vi "Create Table LVClass.vi"(0 "PDF Report":refnum<class "PDF Report Class.lvclass">, 1 "Repeat Headers Row":bool=TRUE, 2 "Table columnWidth [ ]":sgl[](array[numeric]), 3 "Table type":T1, 5 "Column Headers 2D [ ]":string[][](array[string]), 7 "Row Headers 1D [ ]":string[](array[string]), 9 "Text Data 2D [ ]":string[][](array[string]), 11 "error in (no error)":errorcluster, 12 "Image to Add [ ]":T2 {"Scale" format="%#_g %"}) -> (4 "PDF Report duplicate":refnum<class "PDF Report Class.lvclass">, 8 "PDF Table":refnum<class "Pdfp Table Class.lvclass">, 15 "error out":errorcluster)   [LabVIEW 2019]
doc: "Version 2.0\nDeveloped by Jean-Marc Simard\nCopyright © 2012, Exaprom Inc.\nAll rights reserved.\nLicense: BSD\n\nWith iTextSharp 4.1.6 (http://itextsharp.sourceforge.net)\nunder Mozilla Public License Version 1.1\n(http://www.mozilla.org/MPL/MPL-1.1.html)"
uses:
  <userlib>/Exaprom PDF/Controls/General Controls/Image to Add [ ].ctl
  <userlib>/Exaprom PDF/Controls/Image Controls/Image Scale.ctl
  <userlib>/Exaprom PDF/LV Class/Pdfp Table Class/Pdfp Table Class.lvclass
  <userlib>/Exaprom PDF/LV Class/PDF Report Class/PDF Report Class.lvclass
  <userlib>/Exaprom PDF/Controls/Table Controls/Table type.ctl
  <userlib>/Exaprom PDF/Controls/Table Controls/Table Custom Titles or data.ctl
  <userlib>/Exaprom PDF/Controls/Table Controls/Table Custom type Titles or Datas.ctl
  <userlib>/Exaprom PDF/Controls/Table Controls/Cell Border iText number.ctl
  <userlib>/Exaprom PDF/Controls/Font Controls/Font complete B.ctl
  <userlib>/Exaprom PDF/Controls/Font Controls/Font size.ctl
  <userlib>/Exaprom PDF/Controls/Font Controls/Font color.ctl
  <userlib>/Exaprom PDF/Controls/Text Controls/Texte alignement.ctl
  <userlib>/Exaprom PDF/Controls/Table Controls/Cell Vertical alignment.ctl
  <userlib>/Exaprom PDF/Controls/Text Controls/Line spacing.ctl
  <userlib>/Exaprom PDF/Controls/Text Controls/Unicode/ASCII or Unicode with Select.ctl
  <userlib>/Exaprom PDF/Controls/Text Controls/Unicode/Character type with Select.ctl
  <userlib>/Exaprom PDF/Controls/Text Controls/Unicode/Writing direction with Select.ctl
  <userlib>/Exaprom PDF/LV Class/Fonts Class/Font Class.lvclass
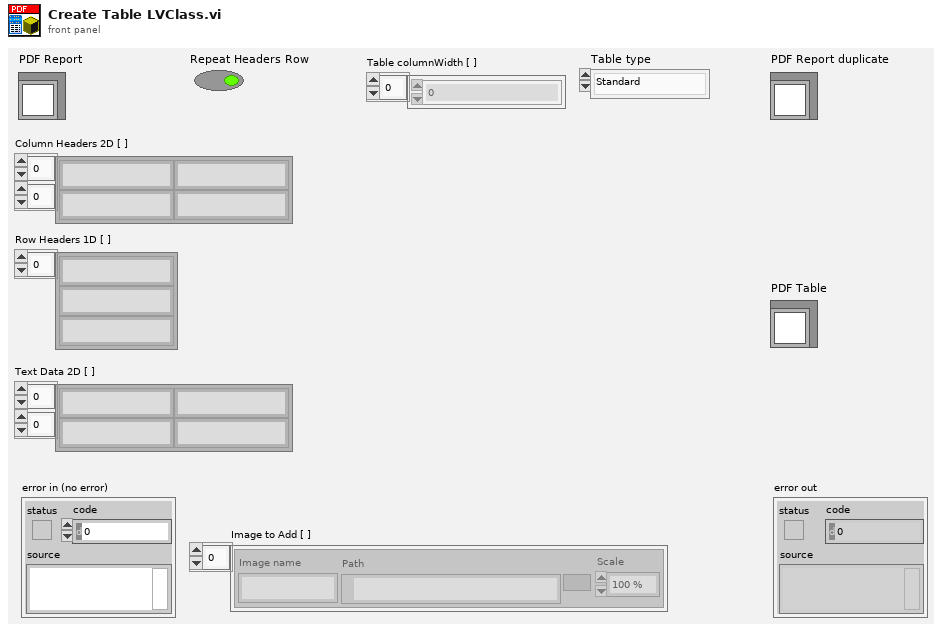
[diagram p1: front panel]
types:
  T1 = typedef "Table type.ctl" = enum16{"Standard", "Customized"}
  T2 = typedef "Image to Add [ ].ctl" = cluster{"Image name":string, "Path":path, "Scale":T3}[]
  T3 = typedef "Image Scale.ctl" = sgl
  T4 = typedef "Table Custom Titles or data.ctl" = cluster{"Titles or datas":T5, "Repeat on each new page?":bool, "Row":cluster{"#":i16, "to #":i16}, "Table columnWidth [ ]":sgl[], "Merge [ ]":cluster{"from":i8, "to":i8}[], "Cell [ ]":cluster{"Cluster 2":cluster{"Cell Border":T6, "Line":cluster{"Thickness":sgl, "Color":u32}, "BG":u32}, "Font":T7, "Align. and LS":cluster{"Horizontal":T10, "Vertical":T11, "Line spacing":T12}}[], "Text 2D":string[][], "ASCII or Unicode":T13}
  T5 = typedef "Table Custom type Titles or Datas.ctl" = enum16{"Title", "Data"}
  T6 = typedef "Cell Border iText number.ctl" = u16
  T7 = typedef "Font complete B.ctl" = cluster{"Name":string, "Size":T8, "Color":T9, "Style":cluster{"Bold":bool, "Italic":bool, "Underline":bool, "Strikeout":bool}, "Embed":bool, "Encoding":string}
  T8 = typedef "Font size.ctl" = sgl
  T9 = typedef "Font color.ctl" = u32
  T10 = typedef "Texte alignement.ctl" = enum16{"Select", "CENTER", "JUSTIFY", "LEFT", "RIGHT"}
  T11 = typedef "Cell Vertical alignment.ctl" = enum16{"TOP", "MIDDLE", "BOTTOM"}
  T12 = typedef "Line spacing.ctl" = enum16{"Select", "1.0", "1.5", "2.0"}
  T13 = typedef "ASCII or Unicode with Select.ctl" = cluster{"Type":T14, "Direction":T15}
  T14 = typedef "Character type with Select.ctl" = enum16{"Select", "ASCII", "Unicode"}
  T15 = typedef "Writing direction with Select.ctl" = enum16{"Select", "Default", "NO BIDI", "LTR", "RTL"}
  T16 = typedef "Font complete cluster.ctl" = cluster{"Name":string, "Size":T8, "Color":T9, "Style":cluster{"Bold":bool, "Italic":bool, "Underline":bool, "Strikeout":bool}, "Type":T17}
  T17 = typedef "Type and encoding.ctl" = cluster{"Type&direction":T18, "Embedded":bool, "Encoding":string}
  T18 = typedef "Type and run direction.ctl" = enum16{"Select", "ASCII", "UTF-16", "UTF-16 (default)", "UTF-16 (LTR)", "UTF-16 (RTL)"}
  T19 = typedef "System Fonts.ctl" = cluster{"Font name [ ]":string[], "Font and file names [ ]":cluster{"Font name":string, "File name":string}[]}
  T20 = typedef "Defaut Paragraphe and Line Spacing.ctl" = cluster{" Aligment":T10, "Line spacing":T12}
  T21 = cluster{"Paragraphe cluster":T20, "Font OUT":T16, "Font Ref":refnum<k24>, "System Fonts":T19}
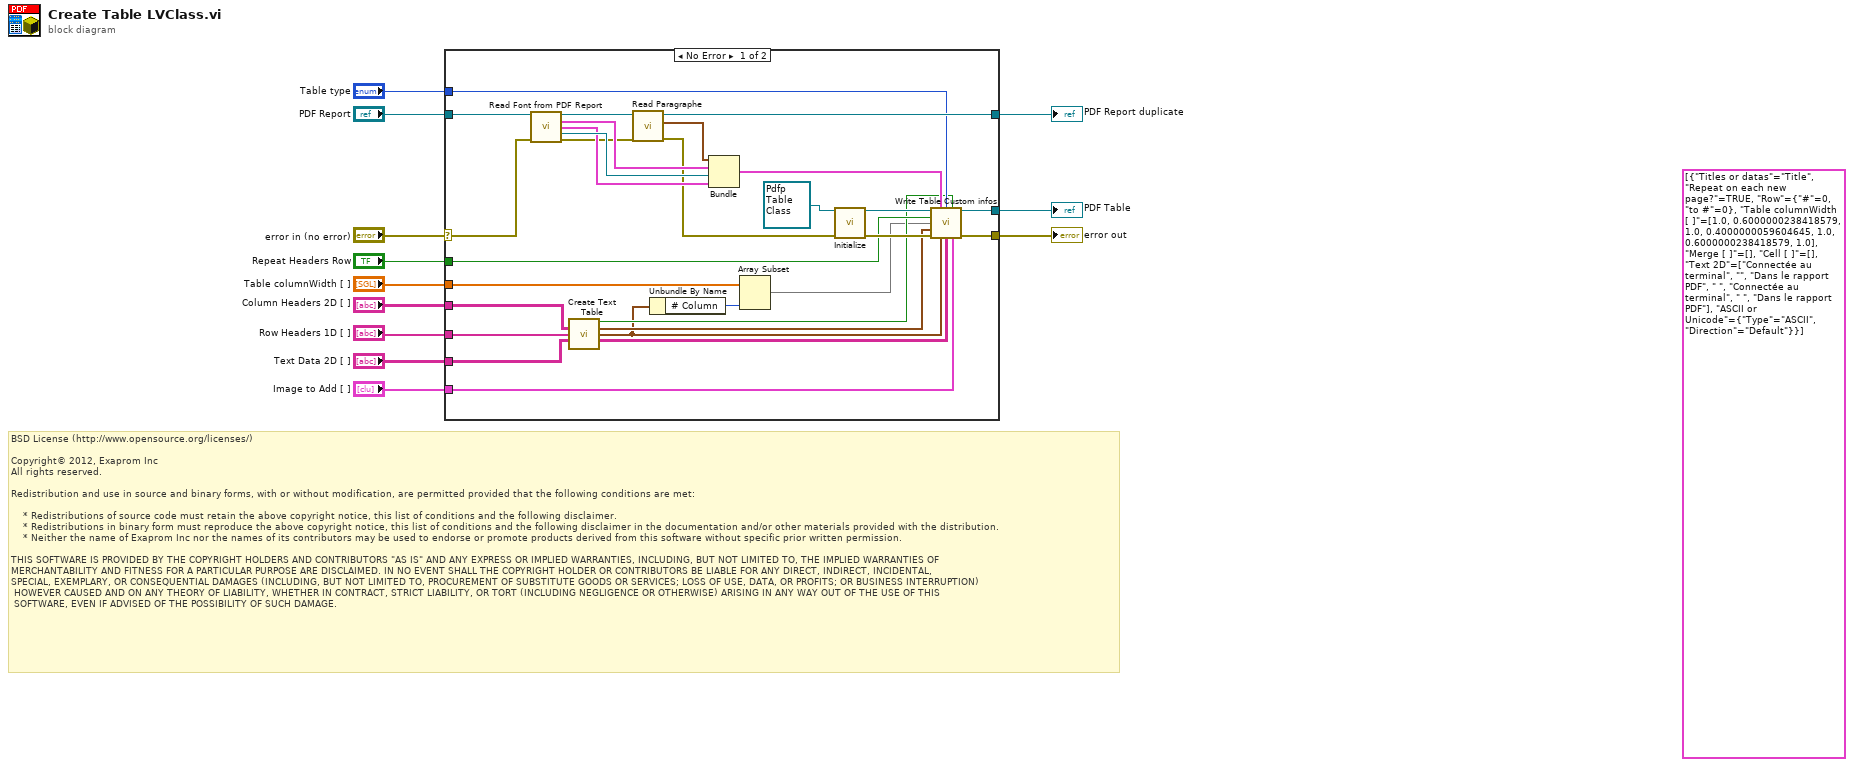
[diagram p0: block diagram]
diagram:
  (unwired) T4[] [{"Titles or datas"=enum."Title", "Repeat on each new page?"=TRUE, "Row"={"#"=0, "to #"=0}, "Table columnWidth [ ]"=[1.0, 0.6, 1.0, 0.4, 1.0, 0.6, 1.0], "Merge [ ]"=[], "Cell [ ]"=[], "Text 2D"=[["Connectée au terminal", "", "Dans le rapport PDF", " ", "Connectée au terminal", " ", "Dans le rapport PDF"]], "ASCII or Unicode"={"Type"=enum."ASCII", "Direction"=enum."Default"}}] ("Table [ ]")
  # "BSD License (http://www.opensource.org/licenses/)\n\nCopyright© 2012, Exaprom Inc\nAll rights reserved.\n\nRedistribution and use in source and binary forms, with or without modification, are permitted provided that the following conditions are met:\n\n    * Redistributions of source code must retain the above copyright notice, this list of conditions and the following disclaimer.\n    * Redistributions in binary form must reproduce the above copyright notice, this list of conditions and the following disclaimer in the documentation and/or other materials provided with the distribution.\n    * Neither the name of Exaprom Inc nor the names of its contributors may be used to endorse or promote products derived from this software without specific prior written permission.\n\nTHIS SOFTWARE IS PROVIDED BY THE COPYRIGHT HOLDERS AND CONTRIBUTORS \"AS IS\" AND ANY EXPRESS OR IMPLIED WARRANTIES, INCLUDING, BUT NOT LIMITED TO, THE IMPLIED WARRANTIES OF \nMERCHANTABILITY AND FITNESS FOR A PARTICULAR PURPOSE ARE DISCLAIMED. IN NO EVENT SHALL THE COPYRIGHT HOLDER OR CONTRIBUTORS BE LIABLE FOR ANY DIRECT, INDIRECT, INCIDENTAL,\nSPECIAL, EXEMPLARY, OR CONSEQUENTIAL DAMAGES (INCLUDING, BUT NOT LIMITED TO, PROCUREMENT OF SUBSTITUTE GOODS OR SERVICES; LOSS OF USE, DATA, OR PROFITS; OR BUSINESS INTERRUPTION)\n HOWEVER CAUSED AND ON ANY THEORY OF LIABILITY, WHETHER IN CONTRACT, STRICT LIABILITY, OR TORT (INCLUDING NEGLIGENCE OR OTHERWISE) ARISING IN ANY WAY OUT OF THE USE OF THIS\n SOFTWARE, EVEN IF ADVISED OF THE POSSIBILITY OF SUCH DAMAGE."
  n1 = case shown="No Error" "error in (no error)" {
    selector: "error in (no error)" -> [w19 w43]
    tunnel: [w40 w43] -> w12
    tunnel: "Repeat Headers Row" -> [w24 _]
    tunnel: "Table columnWidth [ ]" -> [w23 _]
    tunnel: "Image to Add [ ]" -> [w17 _]
    tunnel: [w39 _] -> w7
    tunnel: [w31 w42] -> w6
    tunnel: "PDF Report" -> [w36 w42]
    tunnel: "Table type" -> [w20 _]
    tunnel: "Column Headers 2D [ ]" -> [w27 _]
    tunnel: "Row Headers 1D [ ]" -> [w25 _]
    tunnel: "Text Data 2D [ ]" -> [w26 _]
    frame No Error {
      n2 = call <userlib>:"Read Font from PDF Report.vi"("PDF Report"=w36, "error in (no error)"=w19) -> ("PDF Report duplicate"=w35:refnum<class "PDF Report Class.lvclass">, "Font OUT"=w34:T16, "System Fonts"=w32:T19, "Font Ref"=w33:refnum<k24>, "error out"=w30:errorcluster)  [unwired: 7 in, 2 out]
      n3 = call <userlib>:"Create Text Table.vi"("Column Headers 2D [ ]"=w27, "Row Headers 1D [ ]"=w25, "Text Data 2D [ ]"=w26) -> ("Row Header?"=w16:bool, "Header Column size"=w22:cluster{"# Column":u16, "# Row":u16}, "Table size"=w14:cluster{"# Column":u16, "# Row":u16}, "Text Table 2D [ ]"=w18:string[][])  [unwired: 9 in]
      n4 = call-dynamic "Read Paragraphe.vi"("error in (no error)"=w30, "PDF Report Class in"=w35) -> ("error out"=w29:errorcluster, "Paragraphe cluster"=w28:T20, "PDF Report Class out"=w31:refnum<class "PDF Report Class.lvclass">)  [unwired: 7 in]
      n5 = Unbundle By Name(w14) -> ("# Column"=w13:u16)
      n6 = Bundle("Paragraphe cluster"=w28, "Font OUT"=w34, "Font Ref"=w33, "System Fonts"=w32) -> (w21:T21)  [unwired: 1 out]
      n7 = Array Subset(array=w23, length=w13) -> (w15:sgl[])  [unwired: 1 in]
      n8 = call <userlib>:"Initialize.vi"("PDF Table Class in"=refnum<class "Pdfp Table Class.lvclass"> refnum, "error in (no error)"=w29) -> ("PDF Table Class out"=w38:refnum<class "Pdfp Table Class.lvclass">, "error out"=w37:errorcluster)  [unwired: 12 in]
      n9 = call <userlib>:"Write Table Custom infos.vi"("PDF Table Class.lvclass in"=w38, "Font et paragraph"=w21, "Table type"=w20, "Row Header?"=w16, "Repeat Headers Row"=w24, "Table columnWidth [ ]"=w15, "Header Column size"=w22, "error in (no error)"=w37, "Table size"=w14, "Text Table 2D [ ]"=w18, "Image to Add [ ]"=w17) -> ("PDF Table Class.lvclass out"=w39:refnum<class "Pdfp Table Class.lvclass">, "error out"=w40:errorcluster)  [unwired: 3 in]
    }
    frame Error {
    }
  }
  "error out" <- w12
  "PDF Table" <- w7
  "PDF Report duplicate" <- w6
